vi "IncrementRunCount.vi"(8 "error in (no error)":errorcluster, 10 "Runcount filepath":path, 11 "APU Name":string) -> (0 "error out":errorcluster, 3 "APURunCount out":u32)   [LabVIEW 2018]
uses:
  <vilib>/Utility/config.llb/Read Key (U32).vi
  <vilib>/Utility/config.llb/Write Key (U32).vi
  <vilib>/Utility/config.llb/NI_LVConfig.lvlib
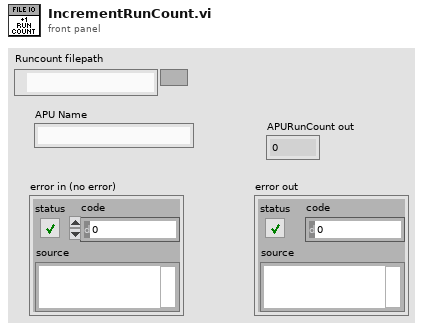
[diagram p1: front panel]
types:
  T1 = typedef "NI_LVConfig.lvlib/Config Data RefNum.ctl" = refnum<k1>
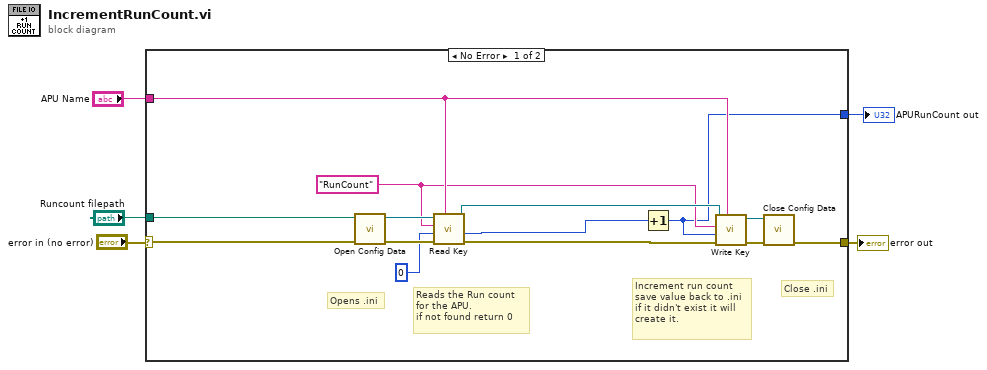
[diagram p0: block diagram]
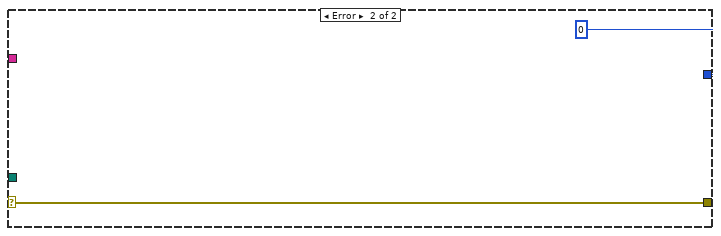
[diagram p2: hidden frame]
diagram:
  n1 = case shown="No Error" "error in (no error)" {
    selector: "error in (no error)" -> [w19 w21]
    tunnel: "APU Name" -> [w14 _]
    tunnel: [w8 w21] -> w4
    tunnel: [w7 u32 0] -> w5
    tunnel: "Runcount filepath" -> [w6 _]
    frame No Error {
      w13 = "RunCount" ("key")
      # "Close .ini"
      # "Opens .ini"
      # "Increment run count\nsave value back to .ini\nif it didn't exist it will \ncreate it."
      # "Reads the Run count \nfor the APU. \nif not found return 0"
      n2 = call <vilib>:"Open Config Data.vi"("error in (no error)"=w19, "configuration file path"=w6) -> ("error out"=w17:errorcluster, "refnum"=w18:T1)  [unwired: 7 in, 1 out]
      n3 = call-poly <vilib>:"Read Key.vi"("section"=w14, "error in (no error)"=w17, "default value"=u32 0, "key"=w13, "refnum"=w18) -> ("error out"=w11:errorcluster, "value"=w12:u32, "refnum out"=w15:T1)  [unwired: 3 in, 1 out]
      n4 = Increment(x=w12) -> (x+1=w7:u32)
      n5 = call-poly <vilib>:"Write Key.vi"("section"=w14, "error in (no error)"=w11, "value"=w7, "key"=w13, "refnum"=w15) -> ("error out"=w9:errorcluster, "refnum out"=w10:T1)  [unwired: 4 in, 1 out]
      n6 = call <vilib>:"Close Config Data.vi"("error in (no error)"=w9, "refnum"=w10) -> ("error out"=w8:errorcluster)  [unwired: 8 in, 1 out]
    }
    frame Error {
    }
  }
  "APURunCount out" <- w5
  "error out" <- w4
